vi "add CRLF.vi"(4 "Flattened Data":string) -> (1 "Data w/CRLF":string)   [LabVIEW 2011]
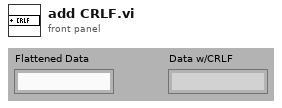
[diagram p1: front panel]
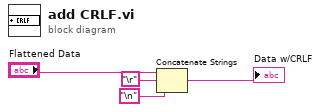
[diagram p0: block diagram]
diagram:
  n1 = Concatenate Strings("Flattened Data", "\r", "\n") -> (→"Data w/CRLF":string)
